vi "JON.vi"(0 "System no.":i32=1 min=1 max=4 step=1, 1 "JoystickID to set":i32[](array[numeric]), 2 "Joystick mode":i32[](array[numeric]), 5 "error in":errorcluster) -> (14 "Controller error":bool, 19 "error out":errorcluster)   [LabVIEW 2020]
doc: "Enables or disables joysticks connected to the controller. Controller error is TRUE if selected system reports an error code which is not 0. Settings will not influence Joystick_Operation_Sample_Program.vi which works with a joystick connected to the host computer.\n\nC-843, C-867, E-861, Mercury, Mercury_GCS: Joystick mode can be 0 (OFF) or 1 (ON). Motion commands like MOV or OSM (if supported) are not allowed when a joystick is active on the axis.\n\nE-709: Only supported if E-709 is used inside C-867K012/K013. Motion commands like MOV are not allowed when a joystick is active on the axis. Joystick mode can be 0 (OFF) or 1 (ON)."
panel:
  # "Enables or disables joysticks connected to the controller."
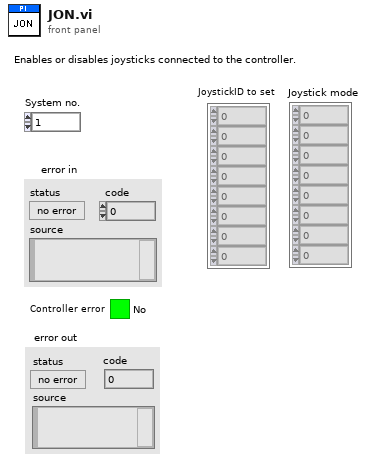
[diagram p1: front panel]
types:
  T1 = enum16{"Disable error check", "Force error check", "Use global settings"}
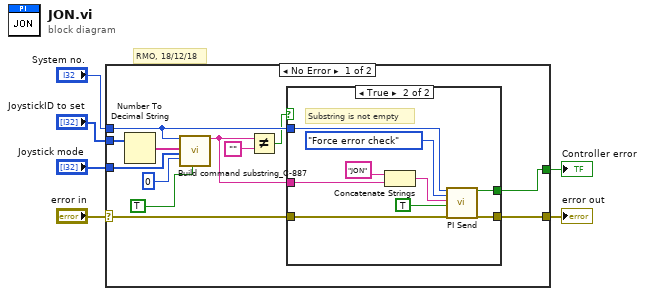
[diagram p0: block diagram]
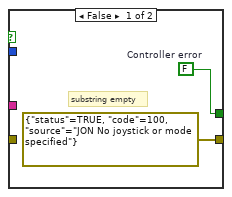
[diagram p2: hidden frame]
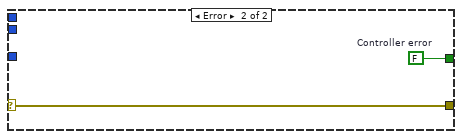
[diagram p3: hidden frame]
diagram:
  # "RMO, 18/12/18"
  n1 = case shown="No Error" "error in" {
    selector: "error in" -> [w8 w31]
    tunnel: [w18 w31] -> w6
    tunnel: "Joystick mode" -> [w15 _]
    tunnel: "System no." -> [w14 _]
    tunnel: "JoystickID to set" -> [w11 _]
    tunnel: [w7 w30] -> w1
    frame No Error {
      n2 = Number To Decimal String(number=w11) -> (decimal integer string=w10:string[])  [unwired: 1 out]
      n3 = call "Build command substring_C-887.vi"("System no."=w14, "Affected axes"=w10, "Parameters"=w15, "No. of digits"=i16 0, "With space?"=TRUE) -> ("Command substring"=w16:string)  [unwired: 2 in, 12 out]
      n4 = Not Equal?(x=w16, y="") -> (x != y?=w13:bool)
      n5 = case shown="True" w13 {
        tunnel: w16 -> [_ w28]
        tunnel: [errorcluster {"status"=TRUE, "code"=100, "source"="JON No joystick or mode specified"} ("error out") w22] -> w18
        tunnel: w8 -> [_ w25]
        tunnel: w14 -> [_ w24]
        tunnel: [w19 w23] -> w7
        frame False {
          w19 = FALSE  # Controller error
          # "substring empty"
        }
        frame True {
          # "Substring is not empty"
          n6 = Concatenate Strings("JON", w28) -> (w26:string)
          n7 = call "PI Send.vi"("System no."=w24, "Error check settings"=T1."Force error check", "String to send"=w26, "Attach termination char.?"=TRUE ("Attach Linefeed?"), "error in"=w25) -> ("Controller error"=w23:bool, "error out"=w22:errorcluster)  [unwired: 1 in, 12 out]
        }
      }
    }
    frame Error {
      w30 = FALSE  # Controller error
    }
  }
  "error out" <- w6
  "Controller error" <- w1
